vi "WriteFeaturesToMap.vi"(8 "error in (no error)":errorcluster, 9 "Map in":T11, 11 "Group":T1) -> (0 "error out":errorcluster, 1 "Map out":T11, 3 "Group out":T1)   [LabVIEW 2017, in "McsaAnalysisLowRate.lvlib"]
uses:
  <vilib>/addons/InsightCM/Devices/Shared/Mcsa/McsaAnalysisLowRate/McsaAnalysisLowRate.lvlib
  <vilib>/addons/PointValueMap/controls/PointMap.ctl
  <vilib>/addons/InsightCM/Devices/Shared/Mcsa/McsaAnalysisLowRate/controls/Group.ctl
  <vilib>/addons/InsightCM/Utilities/Analysis/MCSA/controls/McsaChannel.ctl
  <vilib>/addons/InsightCM/Utilities/Analysis/Shared/controls/Feature.ctl
  <vilib>/addons/InsightCM/Utilities/Analysis/Shared/controls/AmplitudeScale.ctl
  <vilib>/addons/InsightCM/MessageBus/Base/controls/KeyValuePair.ctl
  <vilib>/addons/InsightCM/Utilities/Analysis/MCSA/controls/McsaChannelPhasor.ctl
  <vilib>/addons/InsightCM/Utilities/Analysis/MCSA/controls/McsaMotor.ctl
  <vilib>/addons/InsightCM/Utilities/Analysis/MCSA/controls/MotorCalculationCache.ctl
  <vilib>/addons/Electrical Power/Basic/Measurement/subVIs/basic_Power Value.ctl
  <vilib>/addons/InsightCM/Utilities/Analysis/MCSA/controls/TorqueLoadEfficiency.ctl
  <vilib>/addons/PointValueMap/subVIs/Point_Read_string.vi
  <vilib>/addons/PointValueMap/PointValueMap.lvlib
  <vilib>/addons/InsightCM/Utilities/MCSA/McsaUtilities.lvlib
  <vilib>/addons/InsightCM/Utilities/Analysis/MCSA/McsaAnalysisFunctions.lvlib
  <vilib>/addons/InsightCM/Utilities/Analysis/Shared/AnalysisHelper.lvlib
  <vilib>/addons/Electrical Power/Basic/NI_EP_Basic.lvlib
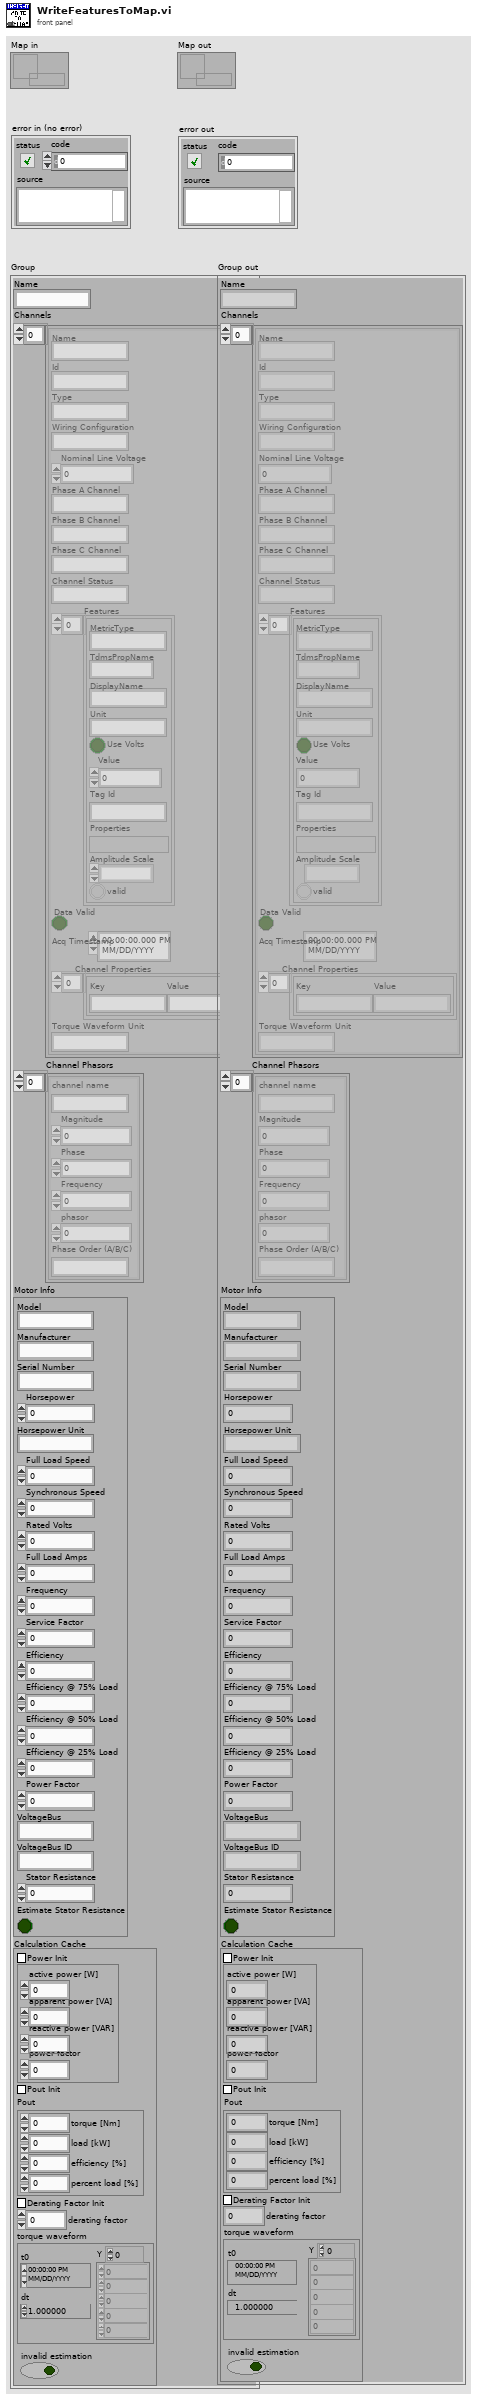
[diagram p1: front panel]
types:
  T1 = typedef "McsaAnalysisLowRate.lvlib/Group.ctl" = cluster{"Name":string, "Channels":T2[], "Channel Phasors":T6[], "Motor Info":T7, "Calculation Cache":T8}
  T2 = typedef "McsaAnalysisFunctions.lvlib/McsaChannel.ctl" = cluster{"Name":string, "Id":string, "Type":string, "Wiring Configuration":string, "Nominal Line Voltage":dbl, "Phase A Channel":string, "Phase B Channel":string, "Phase C Channel":string, "Channel Status":string, "Features":T3[], "Data Valid":bool, "Acq Timestamp":timestamp, "Channel Properties":T5[], "Torque Waveform Unit":string}
  T3 = typedef "AnalysisHelper.lvlib/Feature.ctl" = cluster{"MetricType":string, "TdmsPropName":string, "DisplayName":string, "Unit":string, "Use Volts":bool, "Value":dbl, "Tag Id":string, "Properties":variant, "Amplitude Scale":T4, "valid":bool}
  T4 = typedef "AnalysisHelper.lvlib/AmplitudeScale.ctl" = enum16{"rms", "peak", "pk-pk"}
  T5 = typedef "KeyValuePair.ctl" = cluster{"Key":string, "Value":string}
  T6 = typedef "McsaAnalysisFunctions.lvlib/McsaChannelPhasor.ctl" = cluster{"channel name":string, "Magnitude":dbl, "Phase":dbl, "Frequency":dbl, "phasor":cdb, "Phase Order (A/B/C)":string}
  T7 = typedef "McsaAnalysisFunctions.lvlib/McsaMotor.ctl" = cluster{"Model":string, "Manufacturer":string, "Serial Number":string, "Horsepower":dbl, "Horsepower Unit":string, "Full Load Speed":dbl, "Synchronous Speed":dbl, "Rated Volts":dbl, "Full Load Amps":dbl, "Frequency":dbl, "Service Factor":dbl, "Efficiency":dbl, "Efficiency @ 75% Load":dbl, "Efficiency @ 50% Load":dbl, "Efficiency @ 25% Load":dbl, "Power Factor":dbl, "VoltageBus":string, "VoltageBus ID":string, "Stator Resistance":dbl, "Estimate Stator Resistance":bool}
  T8 = typedef "McsaAnalysisFunctions.lvlib/MotorCalculationCache.ctl" = cluster{"Power Init":bool, "power value":T9, "Pout Init":bool, "Pout":T10, "Derating Factor Init":bool, "derating factor":sgl, "torque waveform":waveform(dbl), "invalid estimation":bool}
  T9 = typedef "NI_EP_Basic.lvlib/basic_Power Value.ctl" = cluster{"active power [W]":dbl, "apparent power [VA]":dbl, "reactive power [VAR]":dbl, "power factor":dbl}
  T10 = typedef "McsaAnalysisFunctions.lvlib/TorqueLoadEfficiency.ctl" = cluster{"torque [Nm]":dbl, "load [kW]":dbl, "efficiency [%]":dbl, "percent load [%]":dbl}
  T11 = typedef "PointValueMap.lvlib/PointMap.ctl" = refnum<data-value>
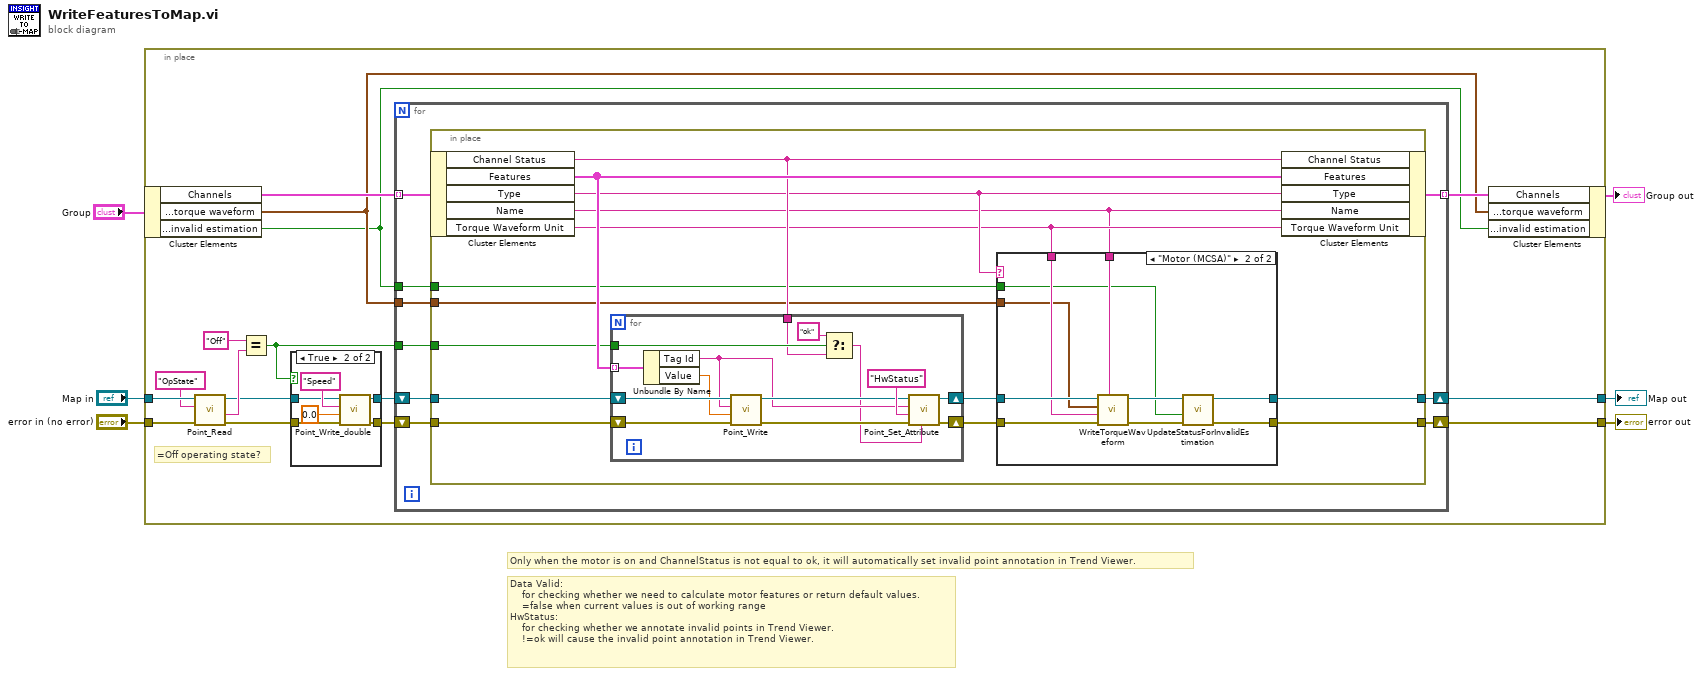
[diagram p0: block diagram]
diagram:
  # "Data Valid: \n    for checking whether we need to calculate motor features or return default values.\n    =false when current values is out of working range\nHwStatus: \n    for checking whether we annotate invalid points in Trend Viewer.\n    !=ok will cause the invalid point annotation in Trend Viewer."
  # "Only when the motor is on and ChannelStatus is not equal to ok, it will automatically set invalid point annotation in Trend Viewer."
  n1 = in-place {
    in-place-border: "Map in" -> [w17]
    in-place-border: "error in (no error)" -> [w18]
    in-place-border: [w19] -> w6
    in-place-border: [w22] -> w3
    # "=Off operating state?"
    n2 = in-place-cluster #1("Group") -> ("Channels"=w21:T2[], "Calculation Cache.torque waveform"=w8:waveform(dbl), "Calculation Cache.invalid estimation"=w7:bool)
    n3 = call-poly <vilib>:"Point_Read.vi"("Error In"=w18, "Tag"="OpState", "Map"=w17) -> ("Error Out"=w13:errorcluster, "Value"=w15:string, "Map Out"=w12:T11)  [unwired: 3 in, 3 out]
    n4 = Equal?(x="Off" ("Tag"), y=w15) -> (x = y?=w9:bool)
    n5 = case shown="True" w9 {
      tunnel: w13 -> [w23 w28]
      tunnel: w12 -> [w24 w27]
      tunnel: [w24 w26] -> w11
      tunnel: [w23 w25] -> w10
      frame False {
      }
      frame True {
        n6 = call <vilib>:"Point_Write_double.vi"("Error In"=w28, "Value"=0.0, "Tag"="Speed", "Map"=w27) -> ("Error Out"=w25:errorcluster, "Map Out"=w26:T11)  [unwired: 6 in]
      }
    }
    n7 = for {
      tunnel: w21 -> [w39] mode=indexing
      shift-right: [w35] -> w22
      shift-left: w11 -> [w38]
      tunnel: [w34] -> w20 mode=indexing
      shift-right: [w36] -> w19
      shift-left: w10 -> [w37]
      tunnel: w9 -> [w33]
      tunnel: w8 -> [w32]
      tunnel: w7 -> [w31]
      n8 = in-place {
        in-place-border: w38 -> [w53]
        in-place-border: w37 -> [w52]
        in-place-border: [w41] -> w36
        in-place-border: [w42] -> w35
        in-place-border: w33 -> [w49]
        in-place-border: w32 -> [w43]
        in-place-border: w31 -> [w40]
        n9 = in-place-cluster #2(w39) -> ("Channel Status"=w50:string, "Features"=w51:T3[], "Type"=w48:string, "Name"=w44:string, "Torque Waveform Unit"=w45:string)
        n10 = for {
          tunnel: w51 -> [w79] mode=indexing
          shift-right: [w71] -> w47
          shift-left: w53 -> [w78]
          shift-right: [w70] -> w46
          shift-left: w52 -> [w77]
          tunnel: w50 -> [w66]
          tunnel: w49 -> [w68]
          n11 = Unbundle By Name(w79) -> ("Tag Id"=w72:string, "Value"=w76:dbl)
          n12 = call-poly <vilib>:"Point_Write.vi"("Error In"=w77, "Value"=w76, "Tag"=w72, "Map"=w78) -> ("Error Out"=w74:errorcluster, "Map Out"=w73:T11)  [unwired: 6 in]
          n13 = Select(t="ok" ("f"), s=w68, f=w66) -> (s? t:f=w69:string)
          n14 = call <vilib>:"Point_Set_Attribute.vi"("Value"=w69, "Error In"=w74, "Attribute"="HwStatus", "Tag"=w72, "Map"=w73) -> ("Error Out"=w70:errorcluster, "Map Out"=w71:T11)  [unwired: 5 in]
        }
        n15 = case shown="\"Motor (MCSA)\"" w48 {
          tunnel: w47 -> [w55 w65]
          tunnel: w46 -> [w54 w64]
          tunnel: w45 -> [_ w63]
          tunnel: w44 -> [_ w62]
          tunnel: w43 -> [_ w61]
          tunnel: [w55 w58] -> w42
          tunnel: [w54 w57] -> w41
          tunnel: w40 -> [_ w56]
          frame Default {
          }
          frame "Motor (MCSA)" {
            n16 = call <vilib>:"WriteTorqueWaveform.vi"("Name"=w62, "error in (no error)"=w64, "Torque Waveform Unit"=w63, "Torque Waveform"=w61, "map in"=w65) -> ("error out"=w59:errorcluster, "map out"=w60:T11)  [unwired: 5 in]
            n17 = call <vilib>:"UpdateStatusForInvalidEstimation.vi"("error in"=w59, "invalid estimation?"=w56, "data map"=w60) -> ("error out"=w57:errorcluster, "data map out"=w58:T11)  [unwired: 7 in]
          }
        }
        n18 = in-place-cluster #2("Channel Status"=w50, "Features"=w51, "Type"=w48, "Name"=w44, "Torque Waveform Unit"=w45) -> (w34:T2)
      }
    }
    n19 = in-place-cluster #1("Channels"=w20, "Calculation Cache.torque waveform"=w8, "Calculation Cache.invalid estimation"=w7) -> (→"Group out":T1)
  }
  "error out" <- w6
  "Map out" <- w3
